vi "Search Tree for Key.vi"(8 "error in":errorcluster, 10 "RegEx In":string, 11 "Tree in":refnum<class "Tree.lvclass">) -> (0 "error out":errorcluster, 1 "Matched Item Values":variant[](array[variant]), 2 "Matched Item Names":string[](array[string]), 3 "Tree out":refnum<class "Tree.lvclass">)   [LabVIEW 2019, in "Tree.lvclass"]
uses:
  Tree.lvclass
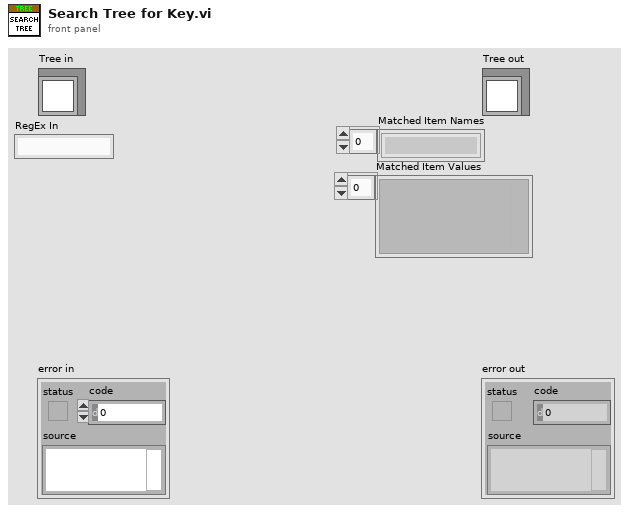
[diagram p1: front panel]
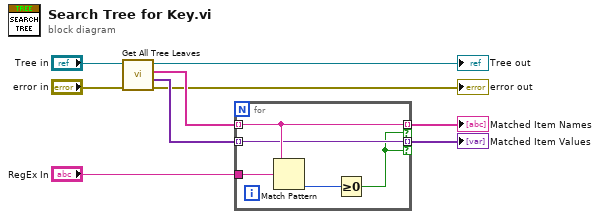
[diagram p0: block diagram]
diagram:
  n1 = call "Get All Tree Leaves.vi"("error in"="error in", "Tree in"="Tree in") -> ("error out"=→"error out":errorcluster, "All Key Values"=w6:variant[], "All Key Names"=w7:string[], "Tree out"=→"Tree out":refnum<class "Tree.lvclass">)  [unwired: 6 in]
  n2 = for {
    tunnel: w7 -> [w12] mode=indexing
    tunnel: "RegEx In" -> [w14]
    tunnel: [w12] -> w5 mode=indexing if=w10
    tunnel: w6 -> [w11] mode=indexing
    tunnel: [w11] -> w4 mode=indexing if=w10
    n3 = Match Pattern(string=w12, regular expression=w14) -> (offset past match=w13:i32)  [unwired: 1 in, 3 out]
    n4 = Greater Or Equal To 0?(x=w13) -> (x >= 0?=w10:bool)
  }
  "Matched Item Names" <- w5
  "Matched Item Values" <- w4
